vi "Add To Fixed Size Array.vi"(10 "New Data":T1[](array[typedef]), 11 "array":T1[](array[typedef])) -> (3 "array out":T1[](array[typedef]))   [LabVIEW 2014, in "SmartPalette.lvlib"]
uses:
  SmartPalette.lvlib
  Controls/GObjectDetail.ctl
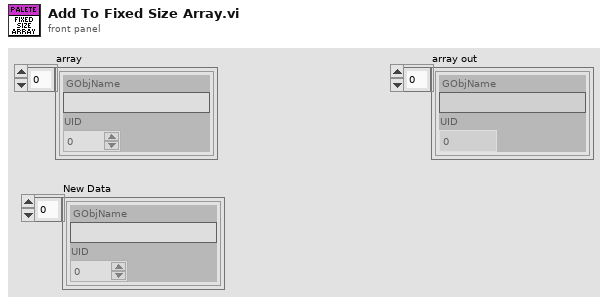
[diagram p1: front panel]
types:
  T1 = typedef "SmartPalette.lvlib/GObjectDetail.ctl" = cluster{"GObjName":string, "UID":i32}
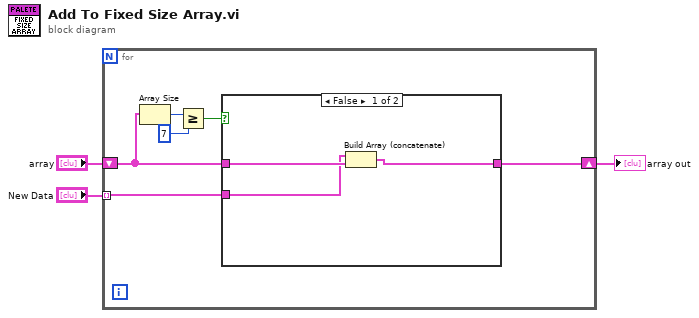
[diagram p0: block diagram]
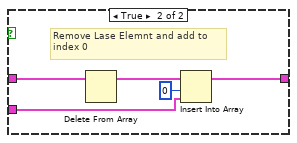
[diagram p2: hidden frame]
diagram:
  n1 = for {
    tunnel: "New Data" -> [w4] mode=indexing
    shift-right: [w5] -> w2
    shift-left: "array" -> [w6]
    n2 = Array Size(array=w6) -> (size(s)=w9:i32)
    n3 = Greater Or Equal?(x=w9, y=7) -> (x >= y?=w7:bool)
    n4 = case shown="False" w7 {
      tunnel: [w12 w16] -> w5
      tunnel: w6 -> [w11 w17]
      tunnel: w4 -> [w10 w13]
      frame False {
        n5 = Build Array (concatenate)(w10, w11) -> (w12:T1[])
      }
      frame True {
        # "Remove Lase Elemnt and add to \nindex 0"
        n6 = Delete From Array(array=w17) -> (array with subset deleted=w15:T1[])  [unwired: 2 in, 1 out]
        n7 = Insert Into Array(array=w15, index=0, new element=w13) -> (w16:T1[])
      }
    }
  }
  "array out" <- w2
